vi "[RE Python] Part 2.vi"(8 "Error In":errorcluster, 10 "Elf Claims":string[][](array[string]), 11 "Fabric":i32[][](array[numeric])) -> (0 "Error Out":errorcluster, 3 "Claim Without Overlap":i32)   [LabVIEW 2019]
doc: "Use the same parsing strategy when building the fabric, but analyze the full fabric. If all of a claim's elements are equivalent to 1, then it has not been overlapped. Return the claim ID of that claim (i.e. the first element of that array in the claim array."
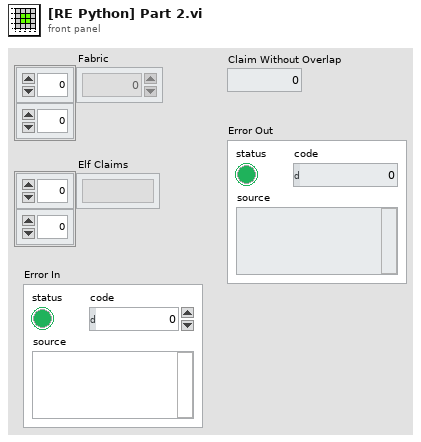
[diagram p1: front panel]
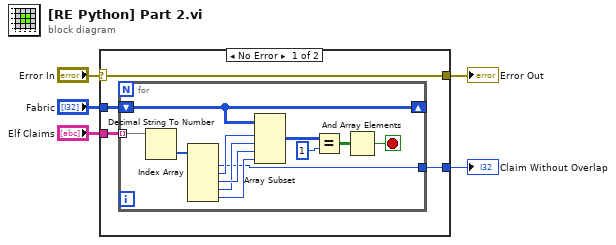
[diagram p0: block diagram]
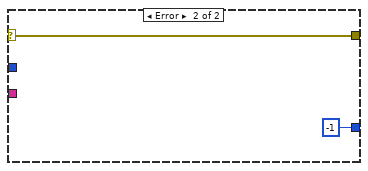
[diagram p2: hidden frame]
diagram:
  n1 = case shown="No Error" "Error In" {
    selector: "Error In" -> [w6 w22]
    tunnel: [w9 -1 ("String")] -> w5
    tunnel: "Elf Claims" -> [w8 _]
    tunnel: "Fabric" -> [w7 _]
    tunnel: [w6 w22] -> w1
    frame No Error {
      n2 = for {
        tunnel: w8 -> [w16] mode=indexing
        shift-right: [w13] -> _
        shift-left: w7 -> [w13]
        tunnel: [w10] -> w9
        stop <- w11 stop-if-true
        n3 = Decimal String To Number(string=w16) -> (number=w17:i32[])  [unwired: 2 in, 1 out]
        n4 = Index Array(array=w17) -> (element #1=w10:i32, element #2=w20:i32, element #3=w21:i32, element #4=w18:i32, element #5=w19:i32)  [unwired: 5 in]
        n5 = Array Subset(array=w13, index (row)=w20, length (row)=w18, index (col)=w21, length (col)=w19) -> (w15:i32[][])
        n6 = Equal?(x=w15, y=1) -> (x = y?=w12:bool[][])
        n7 = And Array Elements(Boolean array=w12) -> (logical AND=w11:bool)
      }
    }
    frame Error {
    }
  }
  "Claim Without Overlap" <- w5
  "Error Out" <- w1
